vi "RunOperation.vi"(10 "Inputs":string[](array[string]), 11 "RunVI in":refnum<class "RunVI.lvclass">) -> (1 "Output/Error messages":string, 2 "CLI Process Return Code":i32, 3 "RunVI out":refnum<class "RunVI.lvclass">)   [LabVIEW 2014, in "RunVI.lvclass"]
uses:
  RunVI.lvclass
  RunVI.lvclass/RunVI.ctl
panel:
  in  "Format Error Output String":string="Error Code : %d\\nError Message : %s\\nAn error occurred while running the %s operation.\\n"
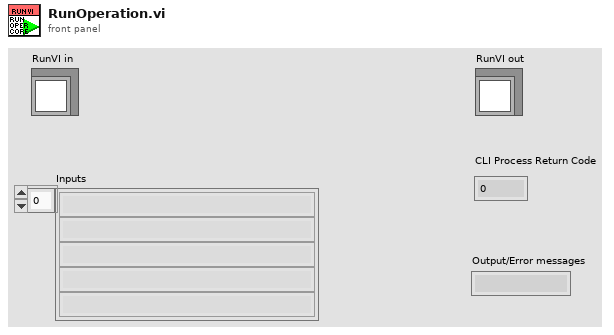
[diagram p1: front panel]
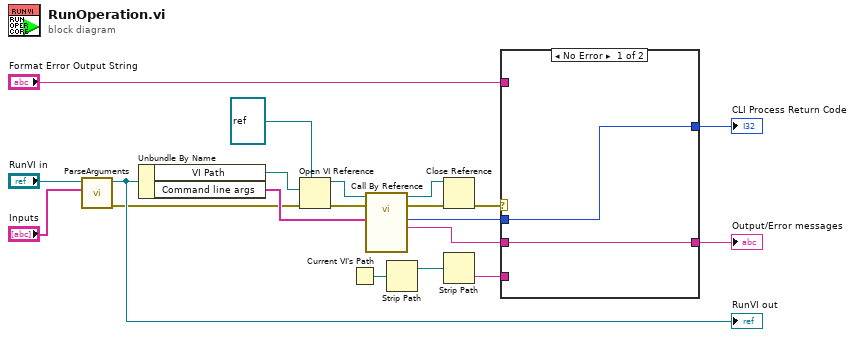
[diagram p0: block diagram]
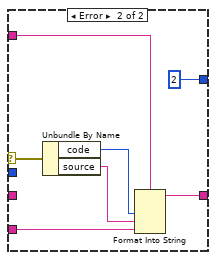
[diagram p2: hidden frame]
diagram:
  n1 = call "ParseArguments.vi"("Inputs"="Inputs", "RunVI in"="RunVI in") -> ("error out"=w12:errorcluster, "RunVI out"=w19:refnum<class "RunVI.lvclass">)  [unwired: 8 in]
  "RunVI out" <- w19
  n2 = Unbundle By Name(w19) -> ("VI Path"=w17:path, "Command line args"=w14:string[])
  n3 = Open VI Reference(type specifier VI Refnum (for type only)=refnum<vi> refnum, vi path=w17, error in (no error)=w12) -> (vi reference=w15:refnum<vi>, error out=w11:errorcluster)  [unwired: 3 in]
  n4 = Current VI's Path() -> (path=w7:path)
  n5 = call-by-ref "?"(reference=w15, error in=w11, "Inputs"=w14) -> (reference out=w13:refnum<vi>, error out=w10:errorcluster, "String"=w1:string, "Numeric"=w4:i32)  [unwired: 9 in]
  n6 = Strip Path(path=w7) -> (stripped path=w6:path)  [unwired: 1 out]
  n7 = Close Reference(reference=w13, error in (no error)=w10) -> (error out=w8:errorcluster)
  n8 = Strip Path(path=w6) -> (name=w5:string)  [unwired: 1 out]
  n9 = case shown="No Error" w8 {
    selector: w8 -> [_ w26]
    tunnel: [w22 w23] -> w2
    tunnel: w1 -> [w22 _]
    tunnel: [w21 2 ("f")] -> w3
    tunnel: "Format Error Output String" -> [_ w28]
    tunnel: w5 -> [_ w27]
    tunnel: w4 -> [w21 _]
    frame No Error {
    }
    frame Error {
      n10 = Unbundle By Name(w26) -> ("code"=w25:i32, "source"=w24:string)
      n11 = Format Into String(format string=w28, w25, w24, w27) -> (resulting string=w23:string)  [unwired: 2 in, 1 out]
    }
  }
  "Output/Error messages" <- w2
  "CLI Process Return Code" <- w3
